vi "Simple GPS Read.vi"(11 "VISA resource name":refnum<visa-resource-name>) -> (0 "Longitude":string, 1 "Latitidue":string, 2 "Time":string, 3 "Current Buffer":string)   [LabVIEW 2009]
uses:
  <vilib>/Instr/_visa.llb/VISA Configure Serial Port (Instr).vi
panel:
  out "x = y?":bool
  in  "stop":bool
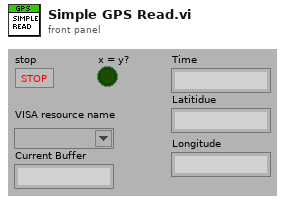
[diagram p1: front panel]
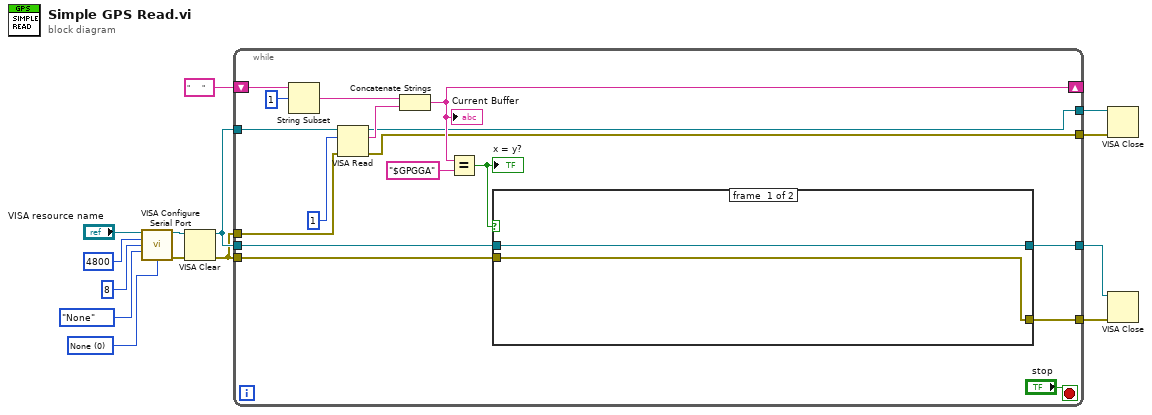
[diagram p0: block diagram]
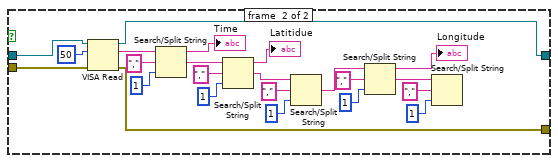
[diagram p2: hidden frame]
diagram:
  w10 = u16 0 items=["None", "XON/XOFF", "RTS/CTS", "XON/XOFF & RTS/CTS", "DTR/DSR", "XON/XOFF & DTR/DSR"] ("flow control (0:none)")
  n1 = call-poly "VISA Configure Serial Port"("VISA resource name"="VISA resource name", "baud rate (9600)"=u32 4800, "data bits (8)"=u16 8, "parity (0:none)"=enum16{"None", "Odd", "Even", "Mark", "Space"}."None", "flow control (0:none)"=w10) -> ("VISA resource name out"=w6:refnum<visa-resource-name>, "error out"=w5:errorcluster)  [unwired: 9 in]
  n2 = VISA Clear(VISA resource name=w6, error in (no error)=w5) -> (VISA resource name out=w4:refnum<visa-resource-name>, error out=w3:errorcluster)
  n3 = while {
    shift-right: [w25] -> _
    shift-left: "      " ("String") -> [w31]
    tunnel: [w23] -> w7
    tunnel: [w22] -> w8
    tunnel: w4 -> [w21]
    tunnel: w3 -> [w20]
    tunnel: w4 -> [w18]
    tunnel: w3 -> [w17]
    tunnel: [w16] -> w2
    tunnel: [w15] -> w1
    stop <- "stop" stop-if-true
    n4 = String Subset(string=w31, offset (0)=1) -> (substring=w27:string)  [unwired: 1 in]
    n5 = VISA Read(VISA resource name=w21, byte count=u32 1, error in (no error)=w20) -> (VISA resource name out=w22:refnum<visa-resource-name>, read buffer=w28:string, error out=w23:errorcluster)  [unwired: 1 out]
    n6 = Concatenate Strings(w27, w28) -> (w25:string)
    "Current Buffer" <- w25
    n7 = Equal?(x=w25, y="$GPGGA") -> (x = y?=w19:bool)
    "x = y?" <- w19
    n8 = case shown="True" w19 {
      tunnel: w18 -> [w33 w56]
      tunnel: w17 -> [w32 w54]
      tunnel: [w33 w37] -> w16
      tunnel: [w32 w36] -> w15
      frame #0 {
      }
      frame #1 {
        n9 = VISA Read(VISA resource name=w56, byte count=u32 50, error in (no error)=w54) -> (VISA resource name out=w37:refnum<visa-resource-name>, read buffer=w53:string, error out=w36:errorcluster)  [unwired: 1 out]
        n10 = Search/Split String(string=w53, search string/char (-)=",", offset (0)=1) -> (substring before match=→"Time":string, match + rest of string=w46:string)  [unwired: 1 out]
        n11 = Search/Split String(string=w46, search string/char (-)=",", offset (0)=1) -> (substring before match=→"Latitidue":string, match + rest of string=w45:string)  [unwired: 1 out]
        n12 = Search/Split String(string=w45, search string/char (-)=",", offset (0)=1) -> (match + rest of string=w42:string)  [unwired: 2 out]
        n13 = Search/Split String(string=w42, search string/char (-)=",", offset (0)=1) -> (substring before match=→"Longitude":string, match + rest of string=w38:string)  [unwired: 1 out]
        n14 = Search/Split String(string=w38, search string/char (-)=",", offset (0)=1) -> ()  [unwired: 3 out]
      }
    }
  }
  n15 = VISA Close(VISA resource name=w8, error in (no error)=w7) -> ()  [unwired: 1 out]
  n16 = VISA Close(VISA resource name=w2, error in (no error)=w1) -> ()  [unwired: 1 out]
